vi "MC5e Terrain_to_String.vi"(11 "Difficult Terrain":i32[](array[numeric])) -> (3 "Difficult Terrain String":string)   [LabVIEW 2020]
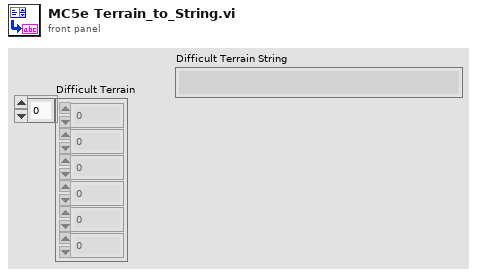
[diagram p1: front panel]
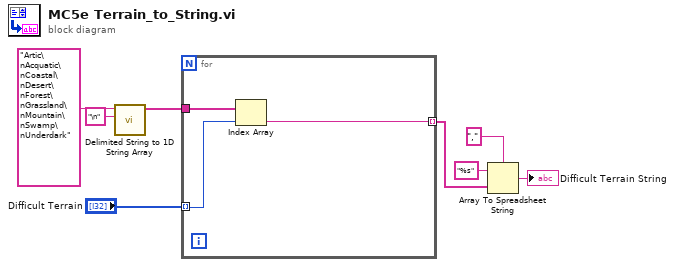
[diagram p0: block diagram]
diagram:
  n1 = call <vilib>:"Delimited String to 1D String Array.vi"("delimiter"="\n", "delimited string"="Artic\nAcquatic\nCoastal\nDesert\nForest\nGrassland\nMountain\nSwamp\nUnderdark" ("input string")) -> ("string array"=w5:string[])  [unwired: 9 in]
  n2 = for {
    tunnel: "Difficult Terrain" -> [w10] mode=indexing
    tunnel: w5 -> [w11]
    tunnel: [w9] -> w4 mode=indexing
    n3 = Index Array(array=w11, index=w10) -> (element=w9:string)
  }
  n4 = Array To Spreadsheet String(delimiter (Tab)=",", array=w4, 3:"%s" ("format string")) -> (spreadsheet string=→"Difficult Terrain String":string)
